vi "Get Channel.vi"(11 "Perform Action on Const Channel Strategy in":refnum<class "Perform Action on Const Channel Strategy.lvclass">) -> (2 "Channel":string, 3 "Perform Action on Const Channel Strategy out":refnum<class "Perform Action on Const Channel Strategy.lvclass">)   [LabVIEW 2024, in "HAL.lvlib" / "Perform Action on Const Channel Strategy.lvclass"]
uses:
  Perform Action on Const Channel Strategy.lvclass
  Perform Action on Const Channel Strategy.lvclass/Perform Action on Const Channel Strategy.ctl
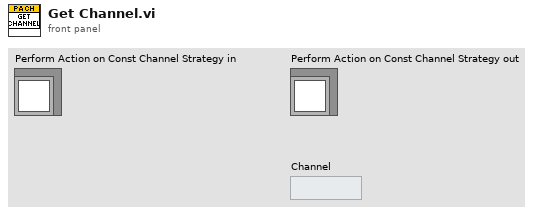
[diagram p1: front panel]
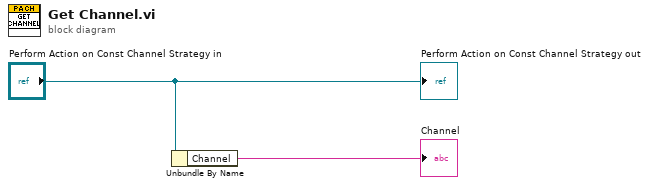
[diagram p0: block diagram]
diagram:
  n1 = Unbundle By Name("Perform Action on Const Channel Strategy in") -> ("Channel"=→"Channel":string)
  "Perform Action on Const Channel Strategy out" <- "Perform Action on Const Channel Strategy in"
